vi "Get DB From Provider.vi"(10 "DBMS Name":string, 11 "Provider":string) -> (3 "database":enum16{"dBase", "Jet", "SQL Server", "Oracle"}(ring))   [LabVIEW 2011]
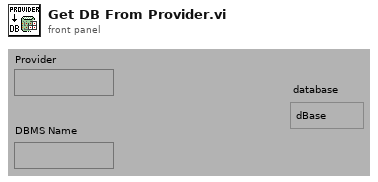
[diagram p1: front panel]
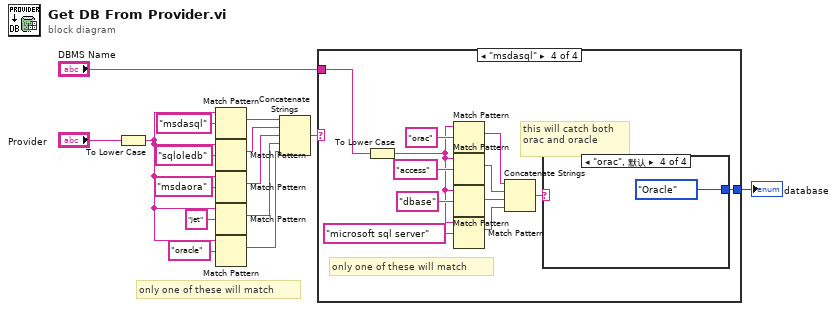
[diagram p0: block diagram]
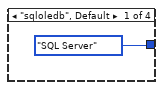
[diagram p2: hidden frame]
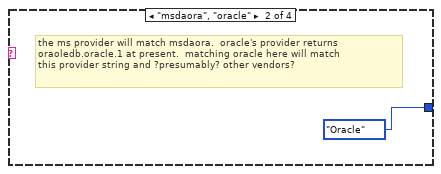
[diagram p3: hidden frame]
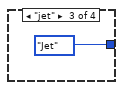
[diagram p4: hidden frame]
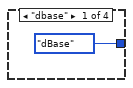
[diagram p5: hidden frame]
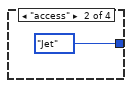
[diagram p6: hidden frame]
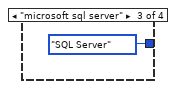
[diagram p7: hidden frame]
diagram:
  # "only one of these will match"
  n1 = To Lower Case(string="Provider") -> (all lower case string=w12:string)
  n2 = Match Pattern(string=w12, regular expression="msdasql") -> (match substring=w5:string)  [unwired: 1 in, 3 out]
  n3 = Match Pattern(string=w12, regular expression="sqloledb") -> (match substring=w9:string)  [unwired: 1 in, 3 out]
  n4 = Match Pattern(string=w12, regular expression="msdaora") -> (match substring=w6:string)  [unwired: 1 in, 3 out]
  n5 = Match Pattern(string=w12, regular expression="jet") -> (match substring=w7:string)  [unwired: 1 in, 3 out]
  n6 = Match Pattern(string=w12, regular expression="oracle" ("string")) -> (match substring=w13:string)  [unwired: 1 in, 3 out]
  n7 = Concatenate Strings(w5, w9, w6, w7, w13) -> (w8:string)
  n8 = case shown="\"msdasql\"" w8 {
    tunnel: [enum16{"dBase", "Jet", "SQL Server", "Oracle"}."SQL Server" ("database") enum16{"dBase", "Jet", "SQL Server", "Oracle"}."Oracle" ("database") enum16{"dBase", "Jet", "SQL Server", "Oracle"}."Jet" ("database") w30] -> w14
    tunnel: "DBMS Name" -> [_ _ _ w19]
    frame "sqloledb", Default {
    }
    frame "msdaora", "oracle" {
      # "the ms provider will match msdaora.  oracle's provider returns\noraoledb.oracle.1 at present.  matching oracle here will match\nthis provider string and ?presumably? other vendors?"
    }
    frame "jet" {
    }
    frame "msdasql" {
      # "this will catch both\norac and oracle"
      # "only one of these will match"
      n9 = To Lower Case(string=w19) -> (all lower case string=w20:string)
      n10 = Match Pattern(string=w20, regular expression="orac") -> (match substring=w25:string)  [unwired: 1 in, 3 out]
      n11 = Match Pattern(string=w20, regular expression="access") -> (match substring=w24:string)  [unwired: 1 in, 3 out]
      n12 = Match Pattern(string=w20, regular expression="dbase") -> (match substring=w23:string)  [unwired: 1 in, 3 out]
      n13 = Match Pattern(string=w20, regular expression="microsoft sql server") -> (match substring=w22:string)  [unwired: 1 in, 3 out]
      n14 = Concatenate Strings(w25, w24, w23, w22) -> (w26:string)
      n15 = case shown="\"orac\", 默认" w26 {
        tunnel: [enum16{"dBase", "Jet", "SQL Server", "Oracle"}."dBase" ("database") enum16{"dBase", "Jet", "SQL Server", "Oracle"}."Jet" ("database") enum16{"dBase", "Jet", "SQL Server", "Oracle"}."SQL Server" ("database") enum16{"dBase", "Jet", "SQL Server", "Oracle"}."Oracle" ("database")] -> w30
        frame "dbase" {
        }
        frame "access" {
        }
        frame "microsoft sql server" {
        }
        frame "orac", Default {
        }
      }
    }
  }
  "database" <- w14
